vi "AutoRoutine1.vi"   [LabVIEW 2020]
doc: "Auto Routine 1 \nSome Parts Not Coded \n\n1. Deposit cone to second tier\n2. Back ip to piece row line\n3. turn 90 degrees rigth\n4. pick up piece\n5. turn left 90 degrees\n6. go to cone box\n7. deposit cone on first tier"
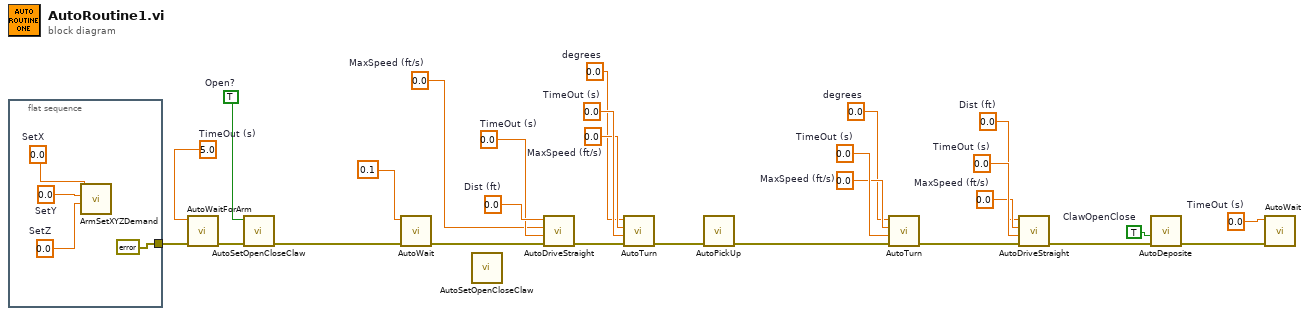
[diagram p0: block diagram]
diagram:
  w1 = 0.0  # degrees
  w2 = 0.0  # MaxSpeed (ft/s)
  w3 = 0.0  # TimeOut (s)
  w4 = 0.0  # Dist (ft)
  w5 = 0.0  # MaxSpeed (ft/s)
  w6 = 0.0  # TimeOut (s)
  w7 = 0.0  # TimeOut (s)
  w8 = TRUE  # ClawOpenClose
  w9 = 0.0  # degrees
  w10 = 0.0  # MaxSpeed (ft/s)
  w11 = 0.0  # TimeOut (s)
  w13 = 0.0  # TimeOut (s)
  w12 = 0.0  # MaxSpeed (ft/s)
  w14 = 0.0  # Dist (ft)
  w15 = 5.0  # TimeOut (s)
  w16 = TRUE  # Open?
  n1 = flat-sequence {
    tunnel: [errorcluster {"status"=FALSE, "code"=0, "source"=""} ("error in (no error)")] -> w21
    frame #0 {
      w28 = 0.0  # SetX
      w29 = 0.0  # SetY
      w30 = 0.0  # SetZ
      n2 = call "ArmSetXYZDemand.vi"("SetZ"=w30, "SetY"=w29, "SetX"=w28) -> ()  [unwired: 9 in]
    }
  }
  n3 = call "AutoWaitForArm.vi"("error in (no error)"=w21, "TimeOut (s)"=w15) -> ("error out"=w20:errorcluster)  [unwired: 9 in]
  n4 = call "AutoSetOpenCloseClaw.vi"("error in (no error)"=w20, "Open?"=w16) -> ("error out"=w19:errorcluster)  [unwired: 9 in]
  n5 = call "AutoWait.vi"("error in (no error)"=w19, "TimeOut (s)"=0.1) -> ("error out"=w18:errorcluster)  [unwired: 9 in]
  n6 = call "AutoSetOpenCloseClaw.vi"() -> ()  [unwired: 11 in, 1 out]
  n7 = call "AutoDriveStraight.vi"("error in (no error)"=w18, "TimeOut (s)"=w13, "MaxSpeed (ft/s)"=w12, "Dist (ft)"=w14) -> ("error out"=w27:errorcluster)  [unwired: 7 in]
  n8 = call "AutoTurn.vi"("error in (no error)"=w27, "TimeOut (s)"=w11, "MaxSpeed (ft/s)"=w10, "degrees"=w9) -> ("error out"=w26:errorcluster)  [unwired: 7 in]
  n9 = call "AutoPickUp.vi"("error in (no error)"=w26) -> ("error out"=w25:errorcluster)  [unwired: 10 in]
  n10 = call "AutoTurn.vi"("error in (no error)"=w25, "TimeOut (s)"=w3, "MaxSpeed (ft/s)"=w2, "degrees"=w1) -> ("error out"=w24:errorcluster)  [unwired: 7 in]
  n11 = call "AutoDriveStraight.vi"("error in (no error)"=w24, "TimeOut (s)"=w6, "MaxSpeed (ft/s)"=w5, "Dist (ft)"=w4) -> ("error out"=w23:errorcluster)  [unwired: 7 in]
  n12 = call "AutoDeposite.vi"("error in (no error)"=w23, "ClawOpenClose"=w8) -> ("error out"=w22:errorcluster)  [unwired: 9 in]
  n13 = call "AutoWait.vi"("error in (no error)"=w22, "TimeOut (s)"=w7) -> ()  [unwired: 9 in, 1 out]
